vi "monitor.vi"() -> ()   [LabVIEW 2015]
panel:
  in  "file (use dialog)":path
  in  "stop":bool
  in  "millisecond multiple":u32=1000
  out "VISA resource name out 2":refnum<visa-resource-name>
  out "read buffer":string
  out "return count 2":u32
  out "error out 2":errorcluster
  in  "byte count":u32
  in  "Limit (A)":dbl
  out "Commands":string
  in  "Voltage (V)":dbl
  out "return count":u32
  in  "VISA resource name":refnum<visa-resource-name>="GPIB0::10::INSTR"
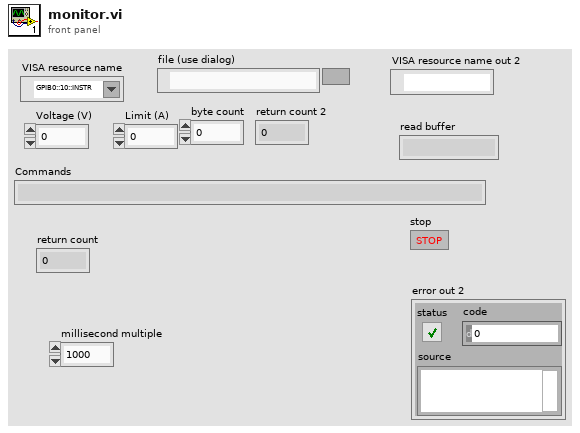
[diagram p1: front panel]
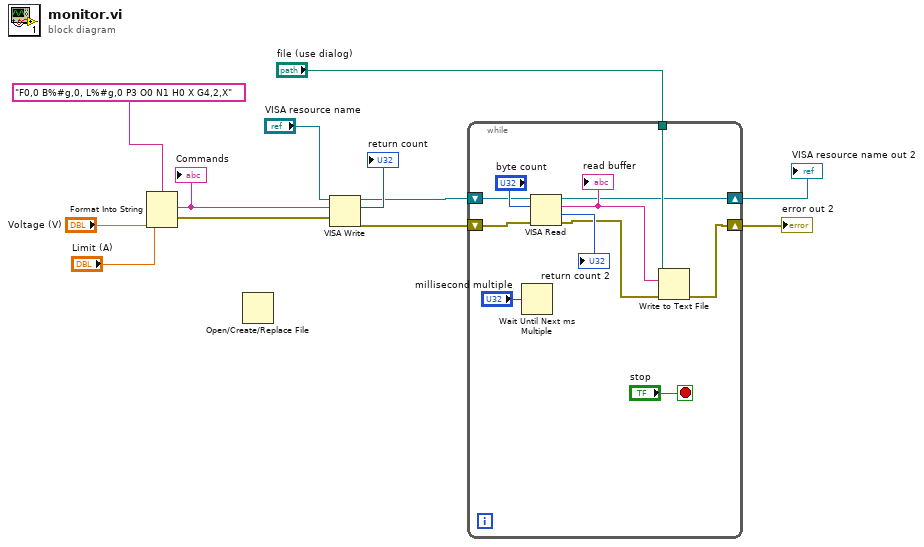
[diagram p0: block diagram]
diagram:
  n1 = Format Into String(format string="F0,0 B%#g,0, L%#g,0 P3 O0 N1 H0 X G4,2,X" ("F0,0X B%f,0,X L%f,0X P3X O0X"), "Voltage (V)", "Limit (A)") -> (resulting string=w8:string, error out=w9:errorcluster)  [unwired: 2 in]
  "Commands" <- w8
  n2 = Open/Create/Replace File() -> ()  [unwired: 6 in, 3 out]
  n3 = VISA Write(VISA resource name="VISA resource name", write buffer=w8, error in (no error)=w9) -> (VISA resource name out=w3:refnum<visa-resource-name>, return count=→"return count":u32, error out=w2:errorcluster)
  n4 = while {
    shift-right: [w13] -> w4
    shift-left: w3 -> [w21]
    shift-right: [w16] -> w5
    shift-left: w2 -> [w20]
    tunnel: "file (use dialog)" -> [w14]
    stop <- "stop" stop-if-true
    n5 = Wait Until Next ms Multiple(millisecond multiple="millisecond multiple") -> ()  [unwired: 1 out]
    n6 = VISA Read(VISA resource name=w21, byte count="byte count", error in (no error)=w20) -> (VISA resource name out=w13:refnum<visa-resource-name>, read buffer=w15:string, return count=→"return count 2":u32, error out=w17:errorcluster)
    "read buffer" <- w15
    n7 = Write to Text File(file (use dialog)=w14, text=w15, error in=w17) -> (error out=w16:errorcluster)  [unwired: 1 in, 2 out]
  }
  "error out 2" <- w5
  "VISA resource name out 2" <- w4
